vi "User_Database_Modify_Confirm.vi"(8 "error in (no error)":errorcluster caption="Error In", 11 "Last_User_Name":string) -> (0 "error out":errorcluster caption="Error Out", 3 "OK":bool)   [LabVIEW 2020]
uses:
  <vilib>/Utility/error.llb/whitespace.ctl
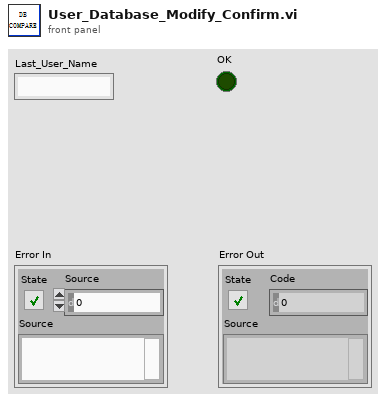
[diagram p1: front panel]
types:
  T1 = cluster{"User_Name":string, "New Password":string, "Confirm Password":string, "User_Right":u16}
  T2 = typedef "whitespace.ctl" = u16
  T3 = typedef "User_Info.ctl" = cluster{"Name":string, "Password":string, "User_Right":u16, "Debuger?":bool, "Manager?":bool, "User_Remember_Name":bool, "User_Remember_PW":bool, "User_Right_String":string, "Null?":bool, "Language":string}
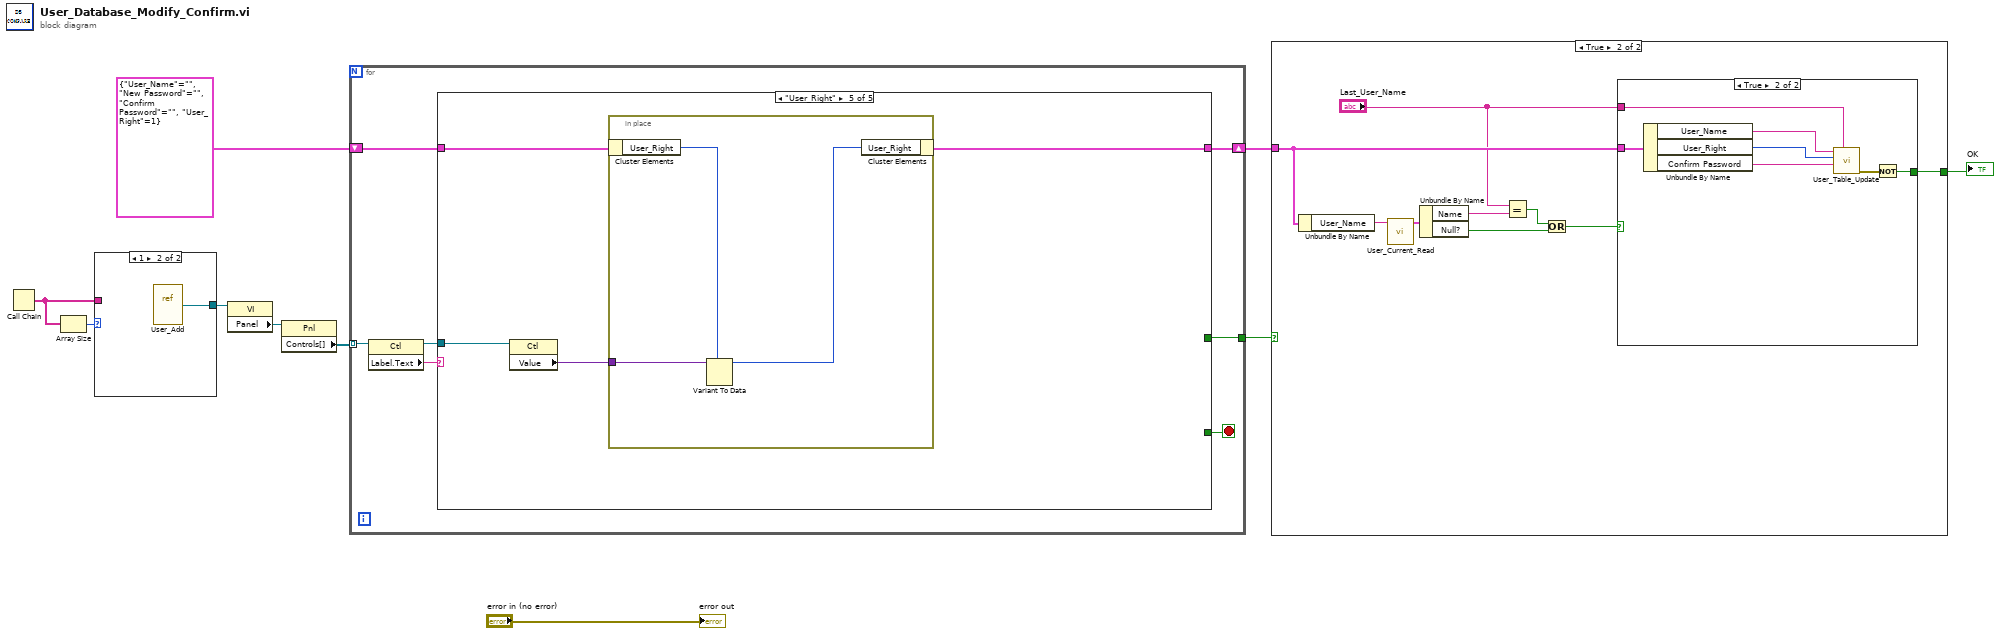
[diagram p0: block diagram]
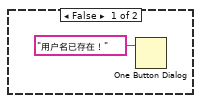
[diagram p3: hidden frame]
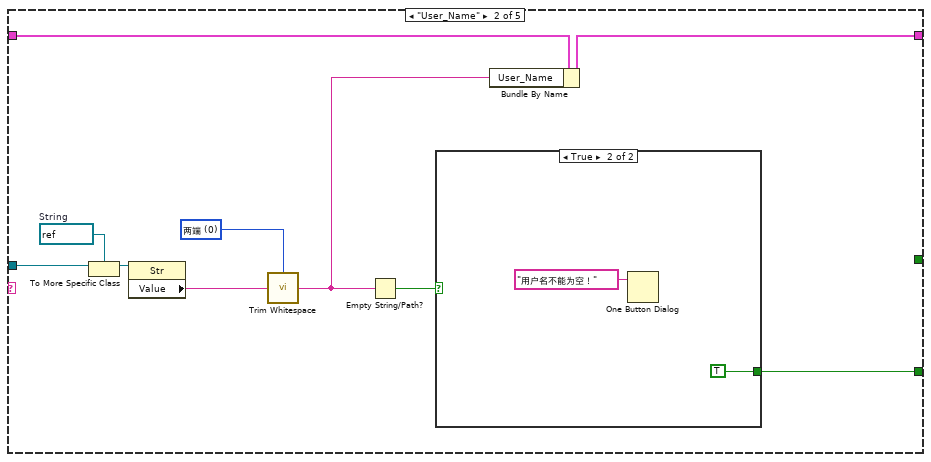
[diagram p5: hidden frame]
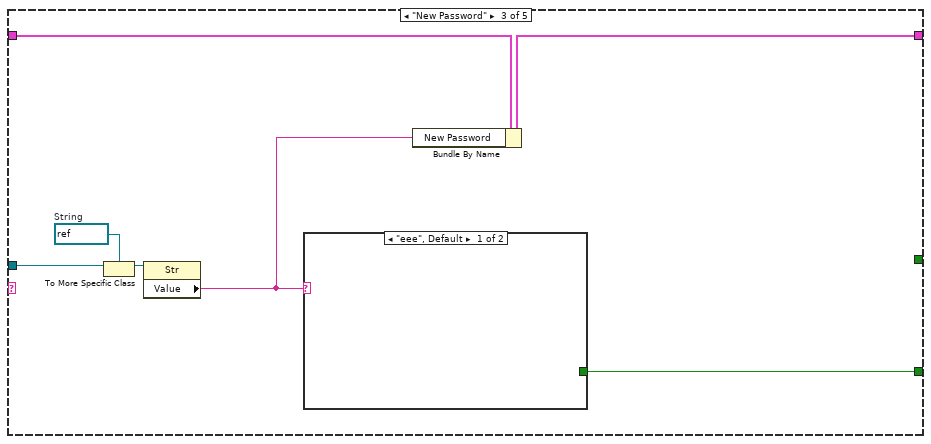
[diagram p7: hidden frame]
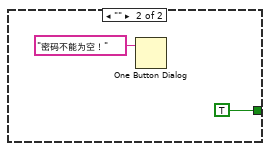
[diagram p8: hidden frame]
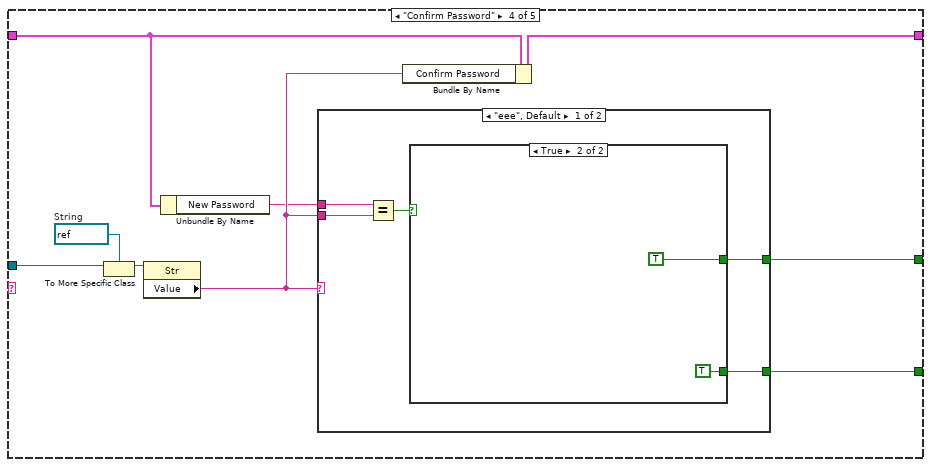
[diagram p9: hidden frame]
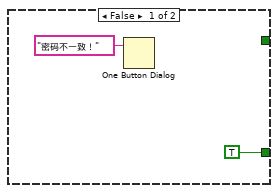
[diagram p10: hidden frame]
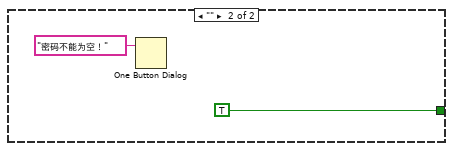
[diagram p11: hidden frame]
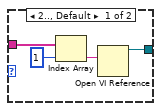
[diagram p12: hidden frame]
diagram:
  n1 = Call Chain() -> (call chain=w7:string[])
  n2 = Array Size(array=w7) -> (size(s)=w8:i32)
  n3 = case shown="1" w8 {
    tunnel: [w12 w15] -> w5
    tunnel: w7 -> [w11 _]
    frame 2.., Default {
      n4 = Index Array(array=w11, index=1 ("索引")) -> (element=w13:string)
      n5 = Open VI Reference(vi path=w13) -> (vi reference=w12:refnum<vi>)  [unwired: 5 in, 1 out]
    }
    frame 1 {
      n6 = vi-ref "User_Add.vi"() -> (w15:refnum<vi>)
    }
  }
  n7 = property class="VI"(reference=w5) -> ("Panel"=w6:refnum<vi>)  [unwired: 1 in, 2 out]
  n8 = property class="Pnl"(reference=w6) -> ("Controls[]"=w9:refnum<vi>[])  [unwired: 1 in, 2 out]
  n9 = for {
    tunnel: w9 -> [w22] mode=indexing
    shift-right: [w17] -> w2
    shift-left: T1 {"User_Name"="", "New Password"="", "Confirm Password"="", "User_Right"=1} -> [w18]
    tunnel: [w16] -> w3
    stop <- w19 stop-if-true
    n10 = property class="Ctl"(reference=w22) -> (reference out=w20:refnum<vi>, "Label.Text"=w21:string)  [unwired: 1 in, 1 out]
    n11 = case shown="\"User_Right\"" w21 {
      tunnel: w20 -> [_ w33 w40 w51 w68]
      tunnel: [_ w28 w39 w50 _] -> w19
      tunnel: w18 -> [w23 w26 w38 w48 w66]
      tunnel: [w23 w25 w36 w49 w65] -> w17
      tunnel: [_ _ _ w45 _] -> w16
      frame "eee", Default {
      }
      frame "User_Name" {
        w30 = T2 0 items=["两端", "字符串首端", "字符串末端"] ("location (both)")
        w32 = refnum<vi> refnum  # String
        n12 = To More Specific Class(target class=w32, reference=w33) -> (specific class reference=w31:refnum<vi>)  [unwired: 1 in, 1 out]
        n13 = property class="Str"(reference=w31) -> ("Value"=w27:string)  [unwired: 1 in, 2 out]
        n14 = call <vilib>:"Trim Whitespace.vi"("string"=w27, "location (both)"=w30) -> ("trimmed string"=w24:string)
        n15 = Empty String/Path?(string/path=w24) -> (empty?=w29:bool)
        n16 = case shown="True" w29 {
          tunnel: [_ TRUE] -> w28
          frame False {
          }
          frame True {
            n17 = One Button Dialog(message="用户名不能为空！" ("消息")) -> ()  [unwired: 1 in, 1 out]
          }
        }
        n18 = Bundle By Name(cluster=w26, "User_Name"=w24) -> (w25:T1)
      }
      frame "New Password" {
        w41 = refnum<vi> refnum  # String
        n19 = To More Specific Class(target class=w41, reference=w40) -> (specific class reference=w42:refnum<vi>)  [unwired: 1 in, 1 out]
        n20 = property class="Str"(reference=w42) -> ("Value"=w37:string)  [unwired: 1 in, 2 out]
        n21 = case shown="\"eee\", Default" w37 {
          tunnel: [_ TRUE] -> w39
          frame "eee", Default {
          }
          frame "" {
            n22 = One Button Dialog(message="密码不能为空！" ("消息")) -> ()  [unwired: 1 in, 1 out]
          }
        }
        n23 = Bundle By Name(cluster=w38, "New Password"=w37) -> (w36:T1)
      }
      frame "Confirm Password" {
        w52 = refnum<vi> refnum  # String
        n24 = To More Specific Class(target class=w52, reference=w51) -> (specific class reference=w53:refnum<vi>)  [unwired: 1 in, 1 out]
        n25 = property class="Str"(reference=w53) -> ("Value"=w47:string)  [unwired: 1 in, 2 out]
        n26 = Unbundle By Name(w48) -> ("New Password"=w46:string)
        n27 = case shown="\"eee\", Default" w47 {
          tunnel: [w55 TRUE] -> w50
          tunnel: w47 -> [w58 _]
          tunnel: w46 -> [w57 _]
          tunnel: [w54 _] -> w45
          frame "eee", Default {
            n28 = Equal?(x=w57, y=w58) -> (x = y?=w56:bool)
            n29 = case shown="True" w56 {
              tunnel: [TRUE TRUE] -> w55
              tunnel: [_ TRUE] -> w54
              frame False {
                n30 = One Button Dialog(message="密码不一致！" ("消息")) -> ()  [unwired: 1 in, 1 out]
              }
              frame True {
              }
            }
          }
          frame "" {
            n31 = One Button Dialog(message="密码不能为空！" ("消息")) -> ()  [unwired: 1 in, 1 out]
          }
        }
        n32 = Bundle By Name(cluster=w48, "Confirm Password"=w47) -> (w49:T1)
      }
      frame "User_Right" {
        n33 = property class="Ctl"(reference=w68) -> ("Value"=w67:variant)  [unwired: 1 in, 2 out]
        n34 = in-place {
          in-place-border: w67 -> [w71]
          n35 = in-place-cluster #1(w66) -> ("User_Right"=w70:u16)
          n36 = Variant To Data(type=w70, Variant=w71) -> (data=w69:u16)  [unwired: 1 in, 1 out]
          n37 = in-place-cluster #1("User_Right"=w69) -> (w65:T1)
        }
      }
    }
  }
  n38 = case shown="True" w3 {
    tunnel: w2 -> [_ w80]
    tunnel: [_ w72] -> w1
    frame False {
    }
    frame True {
      n39 = Unbundle By Name(w80) -> ("User_Name"=w79:string)
      n40 = call "User_Current_Read.vi"("Name"=w79) -> ("User_Info"=w78:T3)  [unwired: 9 in, 1 out]
      n41 = Unbundle By Name(w78) -> ("Name"=w77:string, "Null?"=w75:bool)
      n42 = Equal?(x="Last_User_Name", y=w77) -> (x = y?=w76:bool)
      n43 = Or(x=w76, y=w75) -> (x .or. y?=w74:bool)
      n44 = case shown="True" w74 {
        tunnel: w80 -> [_ w85]
        tunnel: "Last_User_Name" -> [_ w84]
        tunnel: [_ w82] -> w72
        frame False {
          n45 = One Button Dialog(message="用户名已存在！" ("消息")) -> ()  [unwired: 1 in, 1 out]
        }
        frame True {
          n46 = Unbundle By Name(w85) -> ("User_Name"=w88:string, "User_Right"=w87:u16, "Confirm Password"=w86:string)
          n47 = call "User_Table_Update.vi"("Last_User_Name"=w84, "Password"=w86, "User_Right"=w87, "Name"=w88) -> ("error out"=w83:errorcluster)  [unwired: 7 in]
          n48 = Not(x=w83) -> (.not. x?=w82:bool)
        }
      }
    }
  }
  "OK" <- w1
  "error out" <- "error in (no error)"
